vi "IndexCaptor.vi"() -> ()   [LabVIEW 2012]
panel:
  in  "IndexCaptor":i32
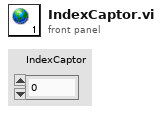
[diagram p1: front panel]
diagram:
